vi "Set VI Ref.vi"(1 "Instrument Prop In":T1 {"Private"."Offset" format="%^_3e"; "Private"."Scale Factors" format="%^_3e"}) -> (0 "Instrument Prop Out":T1 {"Private"."Offset" format="%^_3e"; "Private"."Scale Factors" format="%^_3e"})   [LabVIEW 2019]
uses:
  New NML Data Acq/Sub Controls/Instrument Properties.ctl
  New NML Data Acq/Sub Controls/Public.ctl
  New NML Data Acq/Sub Controls/Private.ctl
  New NML Data Acq/Sub Controls/Instrument Ref.ctl
  New NML Data Acq/Sub Controls/SystemCheckBox-resize.ctl
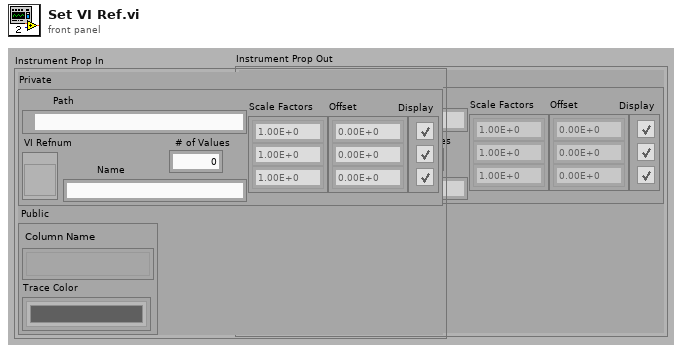
[diagram p1: front panel]
types:
  T1 = typedef "Instrument Properties.ctl" = cluster{"Public":T2, "Private":T3}
  T2 = typedef "Public.ctl" = cluster{"Column Name":string[], "Trace Color":u32[]}
  T3 = typedef "Private.ctl" = cluster{"Path":path, "VI Refnum":T4, "Name":string, "# of Values":i32, "Scale Factors":dbl[], "Display":T5[], "Offset":dbl[]}
  T4 = typedef "Instrument Ref.ctl" = refnum<vi>
  T5 = typedef "SystemCheckBox-resize.ctl" = bool
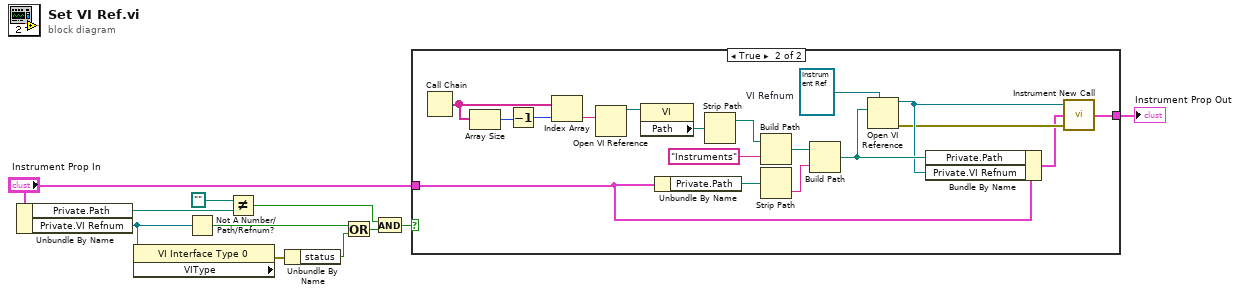
[diagram p0: block diagram]
diagram:
  n1 = Unbundle By Name("Instrument Prop In") -> ("Private.Path"=w4:path, "Private.VI Refnum"=w8:T4)
  n2 = property class="VI Interface Type 0" props=["VIType"](reference=w8) -> (error out=w6:errorcluster)  [unwired: 1 in, 2 out]
  n3 = Not A Number/Path/Refnum?(number/path/refnum=w8) -> (NaN/Path/Refnum?=w9:bool)
  n4 = Not Equal?(x=path "", y=w4) -> (x != y?=w1:bool)
  n5 = Unbundle By Name(w6) -> ("status"=w5:bool)
  n6 = Or(x=w9, y=w5) -> (x .or. y?=w7:bool)
  n7 = And(x=w1, y=w7) -> (x .and. y?=w2:bool)
  n8 = case shown="True" w2 {
    tunnel: "Instrument Prop In" -> [w12 w21]
    tunnel: [w12 w19] -> w10
    frame False {
    }
    frame True {
      w24 = T4 refnum  # VI Refnum
      n9 = Call Chain() -> (call chain=w15:string[])
      n10 = Array Size(array=w15) -> (size(s)=w17:i32)
      n11 = Decrement(x=w17) -> (x-1=w16:i32)
      n12 = Index Array(array=w15, index=w16) -> (element=w14:string)
      n13 = Open VI Reference(vi path=w14) -> (vi reference=w18:refnum<vi>)  [unwired: 5 in, 1 out]
      n14 = property class="VI"(reference=w18) -> ("Path"=w13:path)  [unwired: 1 in, 2 out]
      n15 = Unbundle By Name(w21) -> ("Private.Path"=w26:path)
      n16 = Strip Path(path=w13) -> (stripped path=w27:path)  [unwired: 1 out]
      n17 = Build Path(base path=w27, name or relative path="Instruments") -> (appended path=w29:path)
      n18 = Strip Path(path=w26) -> (name=w25:string)  [unwired: 1 out]
      n19 = Build Path(base path=w29, name or relative path=w25) -> (appended path=w28:path)
      n20 = Open VI Reference(type specifier VI Refnum (for type only)=w24, vi path=w28) -> (vi reference=w23:T4, error out=w22:errorcluster)  [unwired: 4 in]
      n21 = Bundle By Name(cluster=w21, "Private.Path"=w28, "Private.VI Refnum"=w23) -> (w20:T1)
      n22 = call "Instrument New Call.vi"("Error In"=w22, "Instrument Prop In"=w20, "VI Refnum"=w23) -> ("Instrument Prop Out"=w19:T1)  [unwired: 1 in, 1 out]
    }
  }
  "Instrument Prop Out" <- w10
